vi "Orient with Wall.vi"(8 "error in":errorcluster, 10 "Auto Notifiers In":T17, 11 "Auto Refs":T1={"Ultrasonic Forward"={"AIDeviceRef"={"DevStatus"={"status"=FALSE, "code"=0, "source"=""}, "Controller"=enum."Controller 1", "Analog Channel"=enum."Invalid"}, "Scaling factor (V/in)"=0.0098, "Average Bits"=3}, "Ultrasonic Back"={"AIDeviceRef"={"DevStatus"={"status"=FALSE, "code"=0, "source"=""}, "Controller"=enum."Controller 1", "Analog Channel"=enum."Invalid"}, "Scaling factor (V/in)"=0.0098, "Average Bits"=3}, "Strafe Motor"={"DeviceStatus"={"status"=FALSE, "code"=0, "source"=""}, "Type"=enum."PWM", "PWM"={"Controller"=enum."Controller 1", "PWM Channel"=enum."PWM 0", "DeadBand"={"Name"="", "maxPositivePwm"=0, "minPositivePwm"=0, "centerPwm"=0, "maxNegativePwm"=0, "minNegativePwm"=0, "angularRange"=0}}, "CAN"={"Device Number"=0, "Control Mode"=enum."Percent VBus", "Semaphore"=refnum, "Max Vout"=0.0, "TalonSRX Control Mode"=enum."Percent VBus"}, "Invert"=FALSE, "TransformRef"=refnum, "InvTransformRef"=refnum}, "Drive Motors"={"DevStatus"={"status"=FALSE, "code"=0, "source"=""}, "Motors[]"=[], "Square Inputs"=FALSE, "Max Output"=0.0}, "Gyro"={"DevStatus"={"status"=FALSE, "code"=0, "source"=""}, "Analog Module"=enum."Controller 1", "Analog Channel"=enum."Invalid", "Offset"=0.0, "Gain (VoltsPerDegree/Second)"=0.0}} {"Ultrasonic Back"."Average Bits" max=15; "Ultrasonic Forward"."Average Bits" max=15}) -> (0 "error out":errorcluster, 2 "Auto Notifiers Out":T17, 3 "Auto Refs":T1={"Ultrasonic Forward"={"AIDeviceRef"={"DevStatus"={"status"=FALSE, "code"=0, "source"=""}, "Controller"=enum."Controller 1", "Analog Channel"=enum."Invalid"}, "Scaling factor (V/in)"=0.0098, "Average Bits"=3}, "Ultrasonic Back"={"AIDeviceRef"={"DevStatus"={"status"=FALSE, "code"=0, "source"=""}, "Controller"=enum."Controller 1", "Analog Channel"=enum."Invalid"}, "Scaling factor (V/in)"=0.0098, "Average Bits"=3}, "Strafe Motor"={"DeviceStatus"={"status"=FALSE, "code"=0, "source"=""}, "Type"=enum."PWM", "PWM"={"Controller"=enum."Controller 1", "PWM Channel"=enum."PWM 0", "DeadBand"={"Name"="", "maxPositivePwm"=0, "minPositivePwm"=0, "centerPwm"=0, "maxNegativePwm"=0, "minNegativePwm"=0, "angularRange"=0}}, "CAN"={"Device Number"=0, "Control Mode"=enum."Percent VBus", "Semaphore"=refnum, "Max Vout"=0.0, "TalonSRX Control Mode"=enum."Percent VBus"}, "Invert"=FALSE, "TransformRef"=refnum, "InvTransformRef"=refnum}, "Drive Motors"={"DevStatus"={"status"=FALSE, "code"=0, "source"=""}, "Motors[]"=[], "Square Inputs"=FALSE, "Max Output"=0.0}, "Gyro"={"DevStatus"={"status"=FALSE, "code"=0, "source"=""}, "Analog Module"=enum."Controller 1", "Analog Channel"=enum."Invalid", "Offset"=0.0, "Gain (VoltsPerDegree/Second)"=0.0}} {"Ultrasonic Back"."Average Bits" max=15; "Ultrasonic Forward"."Average Bits" max=15})   [LabVIEW 2014]
uses:
  Auto Notifiers.ctl
  Main/Arms/Arm clapper state.ctl
  Main/Arms/Arm State.ctl
  Auto Refs.ctl
  <vilib>/Rock Robotics/WPI/Ultrasonic/WPI_SonarMB1010AnalogDeviceRef.ctl
  <vilib>/Rock Robotics/WPI/AnalogChannel/WPI_AnalogChannelDevRef.ctl
  <vilib>/Rock Robotics/SystemInterfaces/Typedef/FPGA_TypedefAnalogModule.ctl
  <vilib>/Rock Robotics/SystemInterfaces/AI/FPGA_AIChannel.ctl
  <vilib>/Rock Robotics/WPI/MotorControl/WPI_MotorControlDeviceRef.ctl
  <vilib>/Rock Robotics/WPI/MotorControl/WPI_MotorControlType.ctl
  <vilib>/Rock Robotics/SystemInterfaces/Typedef/FPGA_TypedefDigitalModule.ctl
  <vilib>/Rock Robotics/SystemInterfaces/DIO/FPGA_DIOPWMChannel.ctl
  <vilib>/Rock Robotics/WPI/PWM/WPI_PWMDeadband.ctl
  <vilib>/Rock Robotics/WPI/CAN/Jaguar/SubVIs/WPI_CANJaguar_ControlMode.ctl
  <vilib>/Rock Robotics/WPI/CAN/TalonSRX/WPI_CANTalonSRX_APIControlMode.ctl
  <vilib>/Rock Robotics/WPI/PWM/WPI_PWMTransform_ConPane.ctl
  <vilib>/Rock Robotics/WPI/RobotDrive/WPI_RobotDriveDevRef.ctl
  <vilib>/Rock Robotics/WPI/Gyro/WPI_GyroDevRef.ctl
  <vilib>/Rock Robotics/WPI/RobotDrive/WPI_RobotDriveArcadeDrive_Standard(NoSaturation).vi
  <vilib>/Rock Robotics/WPI/Ultrasonic/WPI_SonarSRF04DigitalGetRange.vi
  <vilib>/Rock Robotics/WPI/Ultrasonic/WPI_SonarMB1010AnalogGetRange.vi
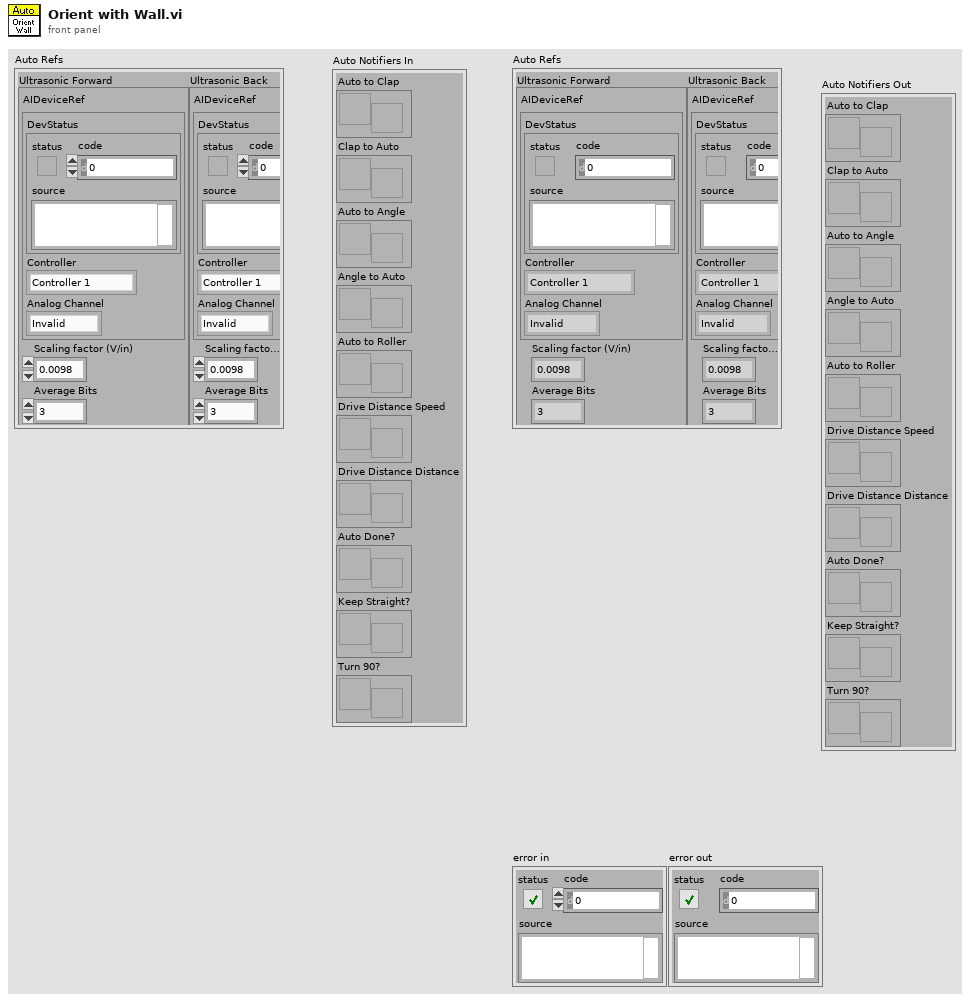
[diagram p1: front panel]
types:
  T1 = typedef "Auto Refs.ctl" = cluster{"Ultrasonic Forward":T2, "Ultrasonic Back":T2, "Strafe Motor":T6, "Drive Motors":T15, "Gyro":T16}
  T2 = typedef "WPI_SonarMB1010AnalogDeviceRef.ctl" = cluster{"AIDeviceRef":T3, "Scaling factor (V/in)":dbl, "Average Bits":u8}
  T3 = typedef "WPI_AnalogChannelDevRef.ctl" = cluster{"DevStatus":errorcluster, "Controller":T4, "Analog Channel":T5}
  T4 = typedef "FPGA_TypedefAnalogModule.ctl" = enum16{"Controller 1"}
  T5 = typedef "FPGA_AIChannel.ctl" = enum8{"AI 0", "AI 1", "AI 2", "AI 3", "AI MXP 0", "AI MXP 1", "AI MXP 2", "AI MXP 3", "Invalid"}
  T6 = typedef "WPI_MotorControlDeviceRef.ctl" = cluster{"DeviceStatus":errorcluster, "Type":T7, "PWM":cluster{"Controller":T8, "PWM Channel":T9, "DeadBand":T10}, "CAN":cluster{"Device Number":u8, "Control Mode":T11, "Semaphore":T12, "Max Vout":dbl, "TalonSRX Control Mode":T13}, "Invert":bool, "TransformRef":T14, "InvTransformRef":T14}
  T7 = typedef "WPI_MotorControlType.ctl" = enum16{"PWM", "CAN", "CANTalonSRX"}
  T8 = typedef "FPGA_TypedefDigitalModule.ctl" = enum16{"Controller 1"}
  T9 = typedef "FPGA_DIOPWMChannel.ctl" = enum8{"PWM 0", "PWM 1", "PWM 2", "PWM 3", "PWM 4", "PWM 5", "PWM 6", "PWM 7", "PWM 8", "PWM 9", "PWM MXP 0", "PWM MXP 1", "PWM MXP 2", "PWM MXP 3", "PWM MXP 4", "PWM MXP 5", "PWM MXP 6", "PWM MXP 7", "PWM MXP 8", "PWM MXP 9", "Invalid"}
  T10 = typedef "WPI_PWMDeadband.ctl" = cluster{"Name":string, "maxPositivePwm":i32, "minPositivePwm":i32, "centerPwm":i32, "maxNegativePwm":i32, "minNegativePwm":i32, "angularRange":u16}
  T11 = typedef "WPI_CANJaguar_ControlMode.ctl" = enum8{"Percent VBus", "Current", "Speed", "Position", "Voltage"}
  T12 = typedef "Semaphore RefNum" = refnum<k1>
  T13 = typedef "WPI_CANTalonSRX_APIControlMode.ctl" = enum8{"Percent VBus", "Speed", "Position", "Slave", "Unchanged / Invalid"}
  T14 = typedef "WPI_PWMTransform_ConPane.ctl" = refnum<vi>
  T15 = typedef "WPI_RobotDriveDevRef.ctl" = cluster{"DevStatus":errorcluster, "Motors[]":T6[], "Square Inputs":bool, "Max Output":dbl}
  T16 = typedef "WPI_GyroDevRef.ctl" = cluster{"DevStatus":errorcluster, "Analog Module":T4, "Analog Channel":T5, "Offset":dbl, "Gain (VoltsPerDegree/Second)":dbl}
  T17 = typedef "Auto Notifiers.ctl" = cluster{"Auto to Clap":refnum<notifier>, "Clap to Auto":refnum<notifier>, "Auto to Angle":refnum<notifier>, "Angle to Auto":refnum<notifier>, "Auto to Roller":refnum<notifier>, "Drive Distance Speed":refnum<notifier>, "Drive Distance Distance":refnum<notifier>, "Auto Done?":refnum<notifier>, "Keep Straight?":refnum<notifier>, "Turn 90?":refnum<notifier>}
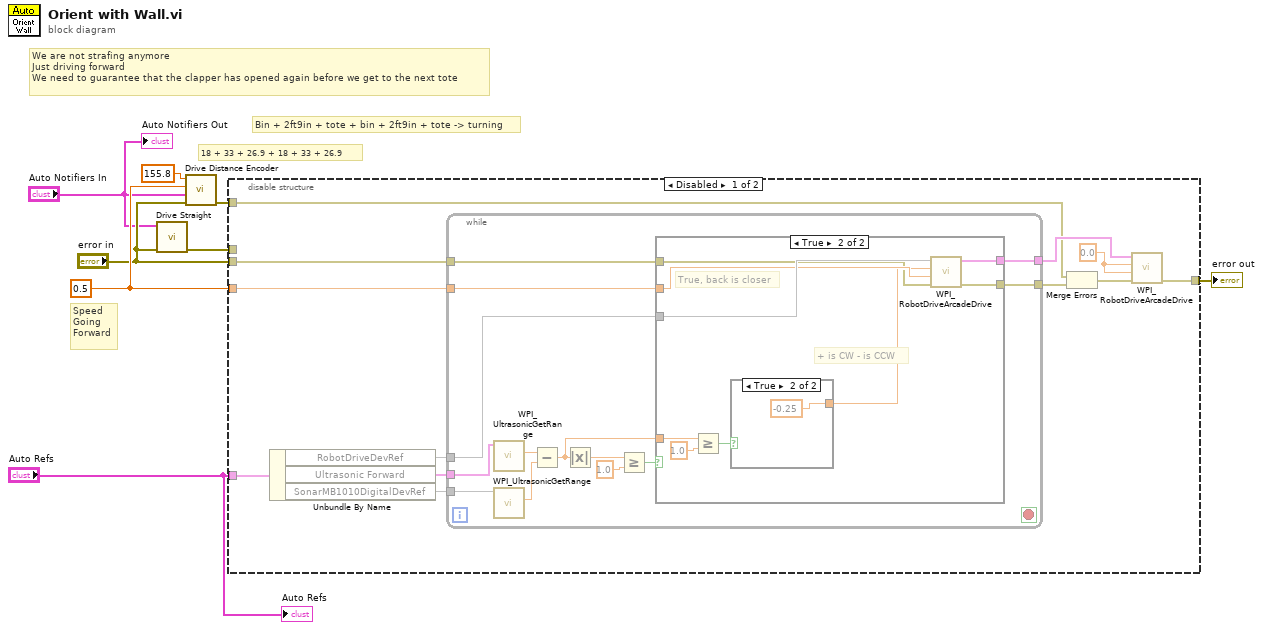
[diagram p0: block diagram]
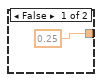
[diagram p3: hidden frame]
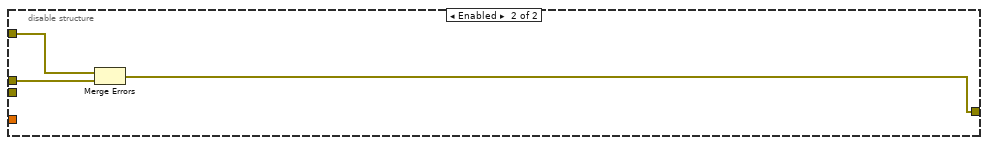
[diagram p4: hidden frame]
diagram:
  w5 = 0.5
  # "Speed\nGoing\nForward"
  # "18 + 33 + 26.9 + 18 + 33 + 26.9"
  # "Bin + 2ft9in + tote + bin + 2ft9in + tote -> turning"
  # "We are not strafing anymore\nJust driving forward\nWe need to guarantee that the clapper has opened again before we get to the next tote"
  n1 = call "Drive Straight.vi"("error in"="error in", "Auto Notifiers In"="Auto Notifiers In") -> ("error out"=w2:errorcluster)  [unwired: 8 in, 1 out]
  n2 = call "Drive Distance Encoder.vi"("error in"="error in", "Auto Notifiers In"="Auto Notifiers In", "Speed"=w5, "Distance (in)"=155.8 ("Distance (inches)")) -> ("error out"=w7:errorcluster)  [unwired: 6 in, 1 out]
  n3 = disable-structure shown="Disabled" {
    disable-tunnel: "Auto Refs" -> [w16 _]
    disable-tunnel: "error in" -> [w13 _]
    disable-tunnel: w7 -> [w12 w47]
    disable-tunnel: [w10 w49] -> w6
    disable-tunnel: w5 -> [w9 _]
    disable-tunnel: w2 -> [_ w48]
    frame Disabled {
      w20 = 0.0 ("X axis value")
      n4 = Unbundle By Name(w16) -> ("RobotDriveDevRef"=w17, "Ultrasonic Forward"=w18:T2, "SonarMB1010DigitalDevRef"=w19)
      n5 = while {
        tunnel: w19 -> [w22]
        tunnel: w18 -> [w23]
        tunnel: w17 -> [w33]
        tunnel: [w32] -> w15
        tunnel: w13 -> [w31]
        tunnel: [w30] -> w14
        tunnel: w9 -> [w29]
        stop <- _ stop-if-true
        n6 = call-poly <vilib>:"WPI_UltrasonicGetRange.vi"("SonarMB1010AnalogDevRef"=w23) -> ("Distance"=w27:dbl)  [unwired: 8 in, 2 out]
        n7 = call-poly <vilib>:"WPI_UltrasonicGetRange.vi"("SonarSRF04DevRef"=w22) -> ("Distance"=w28:dbl)  [unwired: 8 in, 2 out]
        n8 = Subtract(x=w27, y=w28) -> (x-y=w21:dbl)
        n9 = Absolute Value(x=w21) -> (abs(x)=w26:dbl)
        n10 = Greater Or Equal?(x=w26, y=1.0) -> (x >= y?=w24:bool)
        n11 = case shown="True" w24 {
          tunnel: w33 -> [w35 w43]
          tunnel: [w35 w42] -> w32
          tunnel: w31 -> [w34 w36]
          tunnel: [w34 w41] -> w30
          tunnel: w29 -> [_ w39]
          tunnel: w21 -> [_ w38]
          frame False {
          }
          frame True {
            # "+ is CW - is CCW"
            # "True, back is closer"
            n12 = Greater Or Equal?(x=w38, y=1.0) -> (x >= y?=w40:bool)
            n13 = case shown="True" w40 {
              tunnel: [0.25 ("X axis value") -0.25 ("X axis value")] -> w37
              frame False {
              }
              frame True {
              }
            }
            n14 = call-poly <vilib>:"WPI_RobotDriveArcadeDrive.vi"("error in (no error)"=w36, "Y axis value"=w39, "X axis value"=w37, "RobotDriveDevRef"=w43) -> ("error out"=w41:errorcluster, "RobotDriveDevRef"=w42:T15)  [unwired: 5 in, 1 out]
          }
        }
      }
      n15 = Merge Errors(w12, w14) -> (w11:errorcluster)
      n16 = call-poly <vilib>:"WPI_RobotDriveArcadeDrive.vi"("error in (no error)"=w11, "Y axis value"=w20, "X axis value"=w20, "RobotDriveDevRef"=w15) -> ("error out"=w10:errorcluster)  [unwired: 5 in, 2 out]
    }
    frame Enabled {
      n17 = Merge Errors(w47, w48) -> (w49:errorcluster)
    }
  }
  "error out" <- w6
  "Auto Notifiers Out" <- "Auto Notifiers In"
  "Auto Refs" <- "Auto Refs"
